vi "AFT Load Fixed-Point Settings.vi"(8 "error in (no error)":errorcluster, 11 "file path in":path) -> (0 "error out":errorcluster, 2 "fixed-point settings":T1 {"algorithm" items=["LMS"]}, 3 "file path out":path)   [LabVIEW 2017, in "NI_AdaptiveFilter.lvlib"]
doc: "Loads the settings of a fixed-point adaptive filter that you saved to an XML file."
uses:
  <vilib>/addons/Adaptive Filters/NI_AdaptiveFilter.lvlib
  <vilib>/addons/Adaptive Filters/Utilities/AFT Fixed-Point Settings.ctl
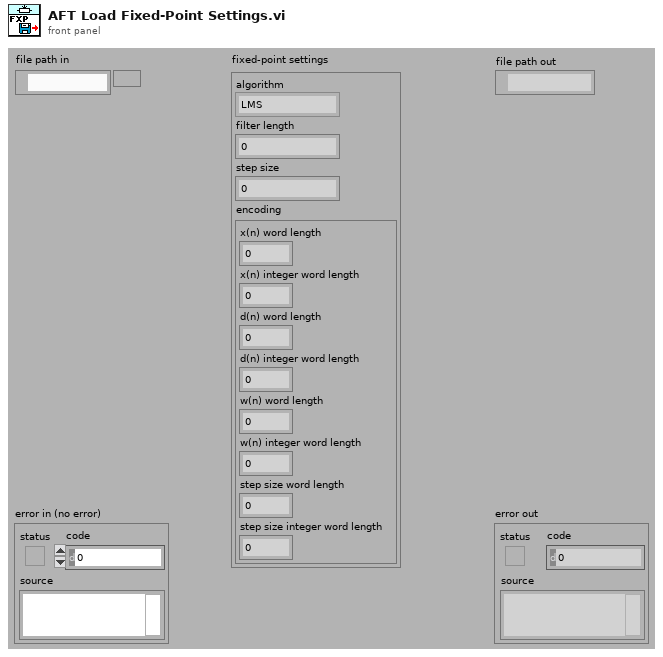
[diagram p1: front panel]
types:
  T1 = typedef "NI_AdaptiveFilter.lvlib/AFT Fixed-Point Settings.ctl" = cluster{"algorithm":u16, "filter length":i32, "step size":dbl, "encoding":cluster{"x(n) word length":i32, "x(n) integer word length":i32, "d(n) word length":i32, "d(n) integer word length":i32, "w(n) word length":i32, "w(n) integer word length":i32, "step size word length":i32, "step size integer word length":i32}}
  T2 = enum16{"open", "open or create", "create or replace", "create", "open (read only)"}
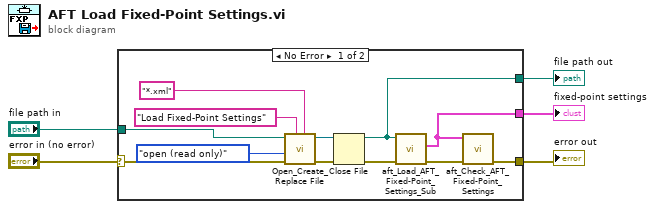
[diagram p0: block diagram]
diagram:
  n1 = case shown="No Error" "error in (no error)" {
    selector: "error in (no error)" -> [w10 w18]
    tunnel: [w16 w18] -> w3
    tunnel: "file path in" -> [w11 _]
    tunnel: [w7 _] -> w1
    tunnel: [w15 _] -> w2
    frame No Error {
      n2 = call <vilib>:"Open_Create_Replace File.vi"("pattern"="*.xml", "prompt"="Load Fixed-Point Settings" ("Prompt"), "error in (no error)"=w10, "function (open:0)"=T2."open (read only)", "file path"=w11) -> ("error out"=w8:errorcluster, "refnum"=w9:refnum<file>)  [unwired: 2 in, 3 out]
      n3 = Close File(refnum=w9, error in=w8) -> (path=w7:path, error out=w6:errorcluster)
      n4 = call <vilib>:"aft_Load_AFT_Fixed-Point_Settings_Sub.vi"("error in (no error)"=w6, "selected path"=w7) -> ("error out"=w17:errorcluster, "AFT fixed-point settings"=w15:T1)  [unwired: 8 out]
      n5 = call <vilib>:"aft_Check_AFT_Fixed-Point_Settings.vi"("error in (no error)"=w17, "AFT fixed-point settings"=w15) -> ("error out"=w16:errorcluster)  [unwired: 9 out]
    }
    frame Error {
    }
  }
  "error out" <- w3
  "fixed-point settings" <- w2
  "file path out" <- w1
